vi "SET_Glyphs [].vi"(8 "error in (no error)":errorcluster, 10 "Glyphs []":T1[](array[typedef]), 11 "Glyph.lvclass in":refnum<class "Glyph.lvclass">) -> (0 "error out":errorcluster, 3 "Glyph.lvclass out":refnum<class "Glyph.lvclass">)   [LabVIEW 2020, in "Glyph.lvclass"]
uses:
  Glyph.lvclass
  Glyph.lvclass/Glyph.ctl
  vi.lib/LabVIEW Icon API/lv_icon/Controls/Graphic.ctl
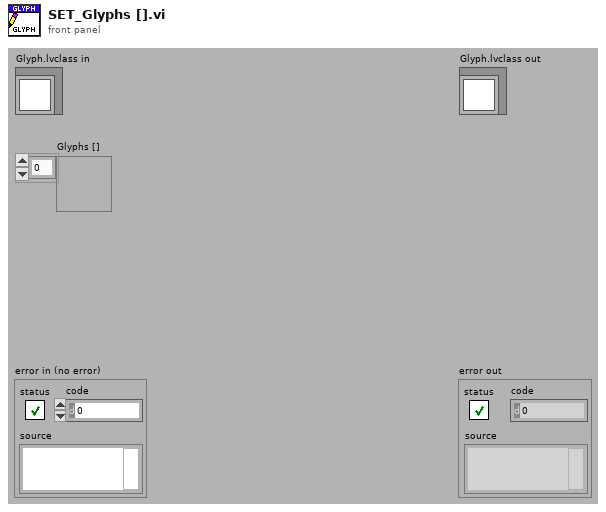
[diagram p1: front panel]
types:
  T1 = typedef "Graphic.ctl" = cluster{"Rectangle":cluster{"left":i16, "top":i16, "right":i16, "bottom":i16}, "Path":path, "Image":picture, "Filter":string, "FileName":string}
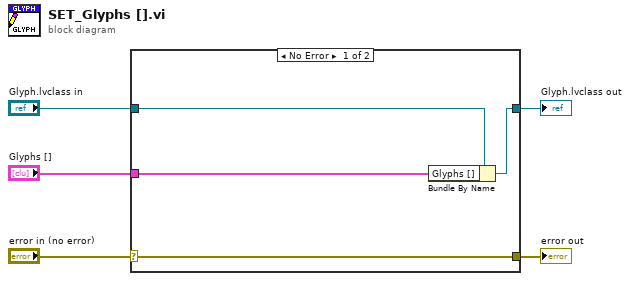
[diagram p0: block diagram]
diagram:
  n1 = case shown="No Error" "error in (no error)" {
    selector: "error in (no error)" -> [w9 w10]
    tunnel: [w9 w10] -> w4
    tunnel: [w7 w11] -> w2
    tunnel: "Glyph.lvclass in" -> [w8 w11]
    tunnel: "Glyphs []" -> [w6 _]
    frame No Error {
      n2 = Bundle By Name(cluster=w8, "Glyphs []"=w6) -> (w7:refnum<class "Glyph.lvclass">)
    }
    frame Error {
    }
  }
  "error out" <- w4
  "Glyph.lvclass out" <- w2
